vi "Read Target Name.vi"(4 "Error In":errorcluster, 7 "Remote Access Commands in":refnum<class "Remote Access Commands.lvclass">) -> (0 "Error Out":errorcluster, 2 "Target Name":string, 3 "Remote Access Commands out":refnum<class "Remote Access Commands.lvclass">)   [LabVIEW 2015, in "Startup Processes.lvlib" / "Remote Access Commands.lvclass"]
uses:
  Remote Access Commands.lvclass
  Remote Access Commands.lvclass/Remote Access Commands.ctl
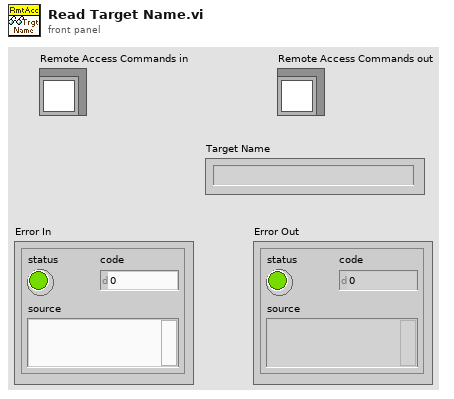
[diagram p1: front panel]
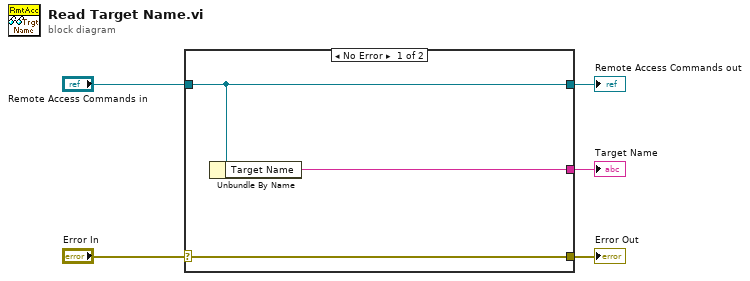
[diagram p0: block diagram]
diagram:
  n1 = case shown="No Error" "Error In" {
    selector: "Error In" -> [w8 w9]
    tunnel: [w8 w9] -> w4
    tunnel: [w7 w10] -> w2
    tunnel: "Remote Access Commands in" -> [w7 w10]
    tunnel: [w6 _] -> w1
    frame No Error {
      n2 = Unbundle By Name(w7) -> ("Target Name"=w6:string)
    }
    frame Error {
    }
  }
  "Error Out" <- w4
  "Remote Access Commands out" <- w2
  "Target Name" <- w1
